vi "BRig_dataBlock_c_BTPR.vi"() -> (2 "output_c_BTPR":i32)   [LabVIEW 2014]
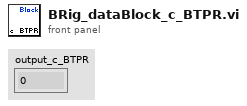
[diagram p1: front panel]
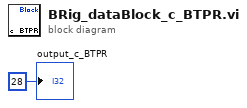
[diagram p0: block diagram]
diagram:
  "output_c_BTPR" <- 28 ("output_iBlock")
